vi "BusInOut.vi"(9 "Existing Obj Name":string, 10 "pins":string[](array[string]), 11 "mbed_LVLibrary.lvlib:mbed.lvclass":refnum<class "mbed.lvclass">) -> (1 "Assigned Name":string, 3 "BusInOut.lvclass 2":refnum<class "BusInOut.lvclass">)   [LabVIEW 2011, in "mbed_LVLibrary.lvlib" / "BusInOut.lvclass"]
uses:
  BusInOut.lvclass
  Transport Mechanisms/mbed/mbed.lvclass
  BusInOut.lvclass/BusInOut.ctl
  <vilib>/regexp/Match Regular Expression.xnode
panel:
  out "error out":errorcluster
  in  "error in (no error)":errorcluster
  in  "BusInOut.lvclass":refnum<class "BusInOut.lvclass">
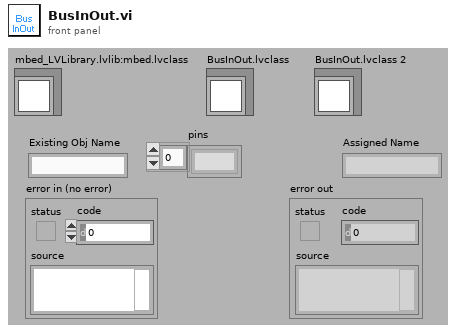
[diagram p1: front panel]
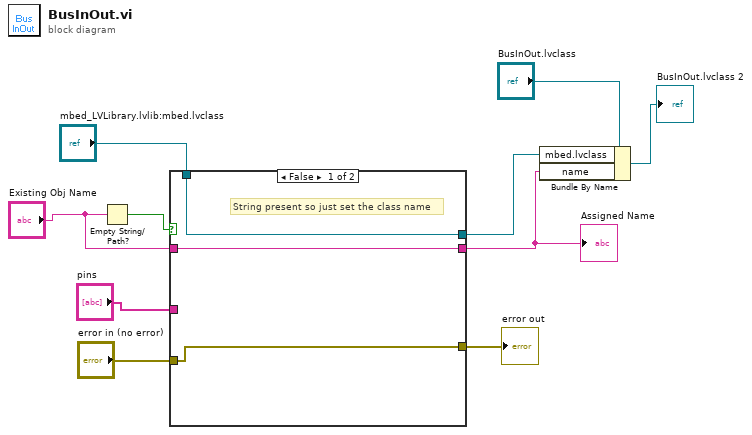
[diagram p0: block diagram]
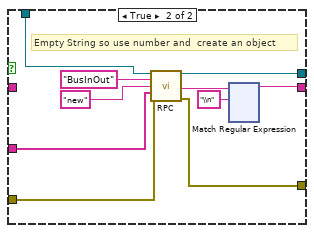
[diagram p2: hidden frame]
diagram:
  n1 = Empty String/Path?(string/path="Existing Obj Name") -> (empty?=w8:bool)
  n2 = case shown="False" w8 {
    tunnel: "Existing Obj Name" -> [w13 _]
    tunnel: [w13 w19] -> w7
    tunnel: "mbed_LVLibrary.lvlib:mbed.lvclass" -> [w12 w23]
    tunnel: [w12 w20] -> w9
    tunnel: "pins" -> [_ w16]
    tunnel: "error in (no error)" -> [w11 w15]
    tunnel: [w11 w14] -> w2
    frame False {
      # "String present so just set the class name"
    }
    frame True {
      # "Empty String so use number and  create an object"
      n3 = call-dynamic "RPC.vi"("mbed in"=w23, "Name"="BusInOut", "method"="new", "Args"=w16, "error in (no error)"=w15) -> ("mbed out"=w20:refnum<class "mbed.lvclass">, "RPC Result"=w18:string, "error out"=w14:errorcluster)  [unwired: 8 in]
      n4 = xnode "Match Regular Expression"("input string"=w18, "regular expression"="\\n") -> ("before match"=w19:string)  [unwired: 4 in, 4 out]
    }
  }
  "Assigned Name" <- w7
  "error out" <- w2
  n5 = Bundle By Name(cluster="BusInOut.lvclass", "mbed.lvclass"=w9, "name"=w7) -> (→"BusInOut.lvclass 2":refnum<class "BusInOut.lvclass">)
